vi "L0_Sum_File_Appender_NU.vi"(0 "Vin":dbl, 1 "CH":dbl, 2 "Att":dbl, 3 "IbClip":dbl=63.0, 4 "Clip":dbl=1.0, 5 "Vmeas":dbl, 7 "file path":path) -> (17 "appended array":dbl[](array[numeric]), 27 "file path 2":path)   [LabVIEW 2012]
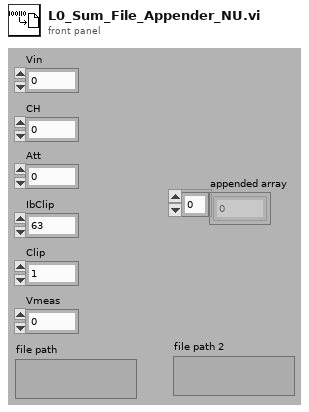
[diagram p1: front panel]
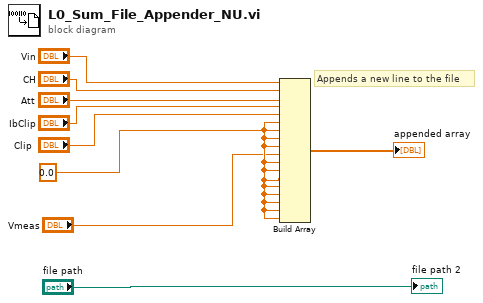
[diagram p0: block diagram]
diagram:
  w9 = 0.0 ("number")
  # "Appends a new line to the file"
  n1 = Build Array("Vin", "CH", "Att", "IbClip", "Clip", w9, w9, w9, w9, "Vmeas", w9, w9, w9, w9, w9, w9, w9, w9) -> (→"appended array":dbl[])
  "file path 2" <- "file path"
